vi "Color Sensor Onshape_Systemlink.vi"() -> ()   [LabVIEW 2020]
uses:
  CEEO/Summer2020/LabVIEWCode/Subs/SystemLink/SL_Subs/SL_XControl.xctl
  <userlib>/Onshape/_SubVI/z did wid and eid.vi
panel:
  in  "stop":bool
  out "Final Color Check":cluster{dbl, dbl, dbl}
  in  "SystemLink":string(xcontrol)="fred"
  out "R Val":dbl
  out "B Val":dbl
  out "G Val":dbl
  out "r Section":string
  out "g Section":string
  out "b Section":string
  out "Sent FeatureScript":string="FeatureScript 1247;\nimport(path : \"onshape/std/geometry.fs\", version : \"1247.0\");\n\nannotation { \"Feature Type Name\" : \"LVFeat1\" }\nexport const myFeature = defineFeature(function(context is Context, id is Id, definition is map)\n    precondition\n    {\n        // Define the parameters of the feature type\n    }\n    {\n        // Define the function's action\n       fEllipsoid(context, id + \"ellipsoid1\", {\n                \"center\" : vector(5, 0, 0) * inch,\n                \"radius\" : vector(3, 3, 3) * inch,\n        });\n\nvar sketch1 = newSketch(context, id + \"sketch1\", {\n                \"sketchPlane\" : qCreatedBy(makeId(\"Top\"), EntityType.FACE)\n        });\n        // Create sketch entities here\n        skRectangle(sketch1, \"rectangle1\", {\n                \"firstCorner\" : vector(0, 0) * inch,\n                \"secondCorner\" : vector(3, 4) * inch\n        });\n        \n        skSolve(sketch1);\n    });"
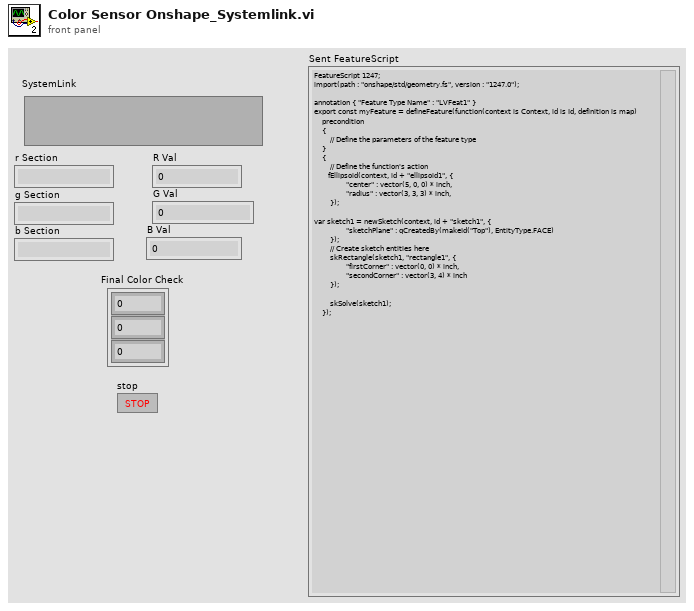
[diagram p1: front panel]
types:
  T1 = cluster{"Point 1":cluster{"y":dbl, "z":dbl, "x":dbl}, "Point 2":cluster{"x":dbl, "y":dbl, "z":dbl}, "Point 3":cluster{"x":dbl, "z":dbl, "y":dbl}}
  T2 = typedef "Cluster.ctl" = cluster{"Date":string, "On-Nonce":string, "eid":string, "wid":string, "did":string, "name":string, "method":string, "Accept":string, "User-Agent":string, "Content-Type":string, "stack":string, "headers":string[], "payload":string, "addition":string, "path":string, "Authorization":string, "secret_key":string, "access_key":string}
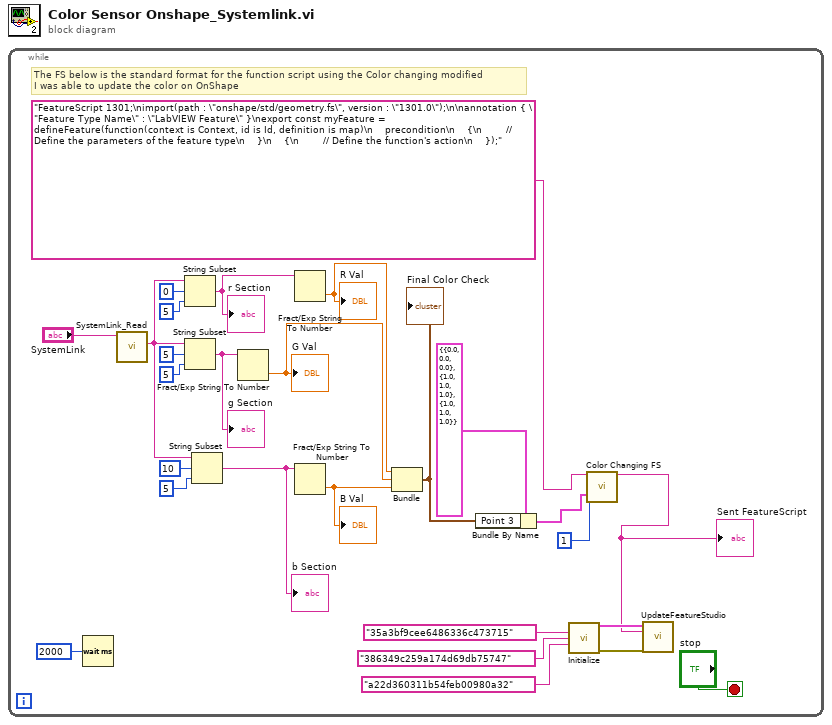
[diagram p0: block diagram]
diagram:
  n1 = while {
    stop <- "stop" stop-if-true
    # "The FS below is the standard format for the function script using the Color changing modified\nI was able to update the color on OnShape"
    n2 = Wait (ms)(milliseconds to wait=u32 2000) -> ()  [unwired: 1 out]
    n3 = call "SystemLink_Read.vi"("SystemLink Tag"="SystemLink") -> ("value"=w8:string)  [unwired: 7 in, 3 out]
    n4 = String Subset(string=w8, offset (0)=0, length (rest)=5 ("length (rest)")) -> (substring=w9:string)
    "r Section" <- w9
    n5 = String Subset(string=w8, offset (0)=5, length (rest)=5 ("length (rest)")) -> (substring=w12:string)
    "g Section" <- w12
    n6 = String Subset(string=w8, offset (0)=10, length (rest)=5 ("length (rest)")) -> (substring=w13:string)
    "b Section" <- w13
    n7 = Fract/Exp String To Number(string=w12) -> (number=w23:dbl)  [unwired: 3 in, 1 out]
    "G Val" <- w23
    n8 = Fract/Exp String To Number(string=w9) -> (number=w24:dbl)  [unwired: 3 in, 1 out]
    "R Val" <- w24
    n9 = Fract/Exp String To Number(string=w13) -> (number=w22:dbl)  [unwired: 3 in, 1 out]
    "B Val" <- w22
    n10 = Bundle(w24, w23, w22) -> (w20:cluster{dbl, dbl, dbl})  [unwired: 1 in]
    "Final Color Check" <- w20
    n11 = Bundle By Name(cluster=T1 {"Point 1"={"y"=0.0, "z"=0.0, "x"=0.0}, "Point 2"={"x"=1.0, "y"=1.0, "z"=1.0}, "Point 3"={"x"=1.0, "z"=1.0, "y"=1.0}} ("Cuboid"), "Point 3"=w20) -> (w3:T1)
    n12 = call-poly <userlib>:"Initialize.vi"("did"="35a3bf9cee6486336c473715", "wid"="386349c259a174d69db75747", "eid"="a22d360311b54feb00980a32") -> ("Device Out"=w6:T2, "error out"=w5:errorcluster)  [unwired: 11 in]
    n13 = call <userlib>:"Color Changing FS.vi"("Feature In"="FeatureScript 1301;\nimport(path : \"onshape/std/geometry.fs\", version : \"1301.0\");\n\nannotation { \"Feature Type Name\" : \"LabVIEW Feature\" }\nexport const myFeature = defineFeature(function(context is Context, id is Id, definition is map)\n    precondition\n    {\n        // Define the parameters of the feature type\n    }\n    {\n        // Define the function's action\n    });", "Cuboid"=w3, "Body #"=1) -> ("Feature Out"=w1:string)  [unwired: 16 in]
    "Sent FeatureScript" <- w1
    n14 = call <userlib>:"UpdateFeatureStudio.vi"("Device In"=w6, "FeatureScript"=w1, "error in"=w5) -> ()  [unwired: 10 in, 3 out]
  }
